vi "Launch Scoring Manager.vi"(8 "error in (no error)":errorcluster, 11 "SOL-Server in":refnum<class "SOL-Server.lvclass">) -> (0 "error out":errorcluster, 3 "SOL-Server out":refnum<class "SOL-Server.lvclass">)   [LabVIEW 2020, in "Summer of LabVIEW.lvlib" / "SOL-Server.lvclass"]
uses:
  SOL-Server.lvclass
  Scoring Manager Async.vi
  SOL-Server.lvclass/SOL-Server.ctl
  SOL-Config/SOL-Config.lvclass
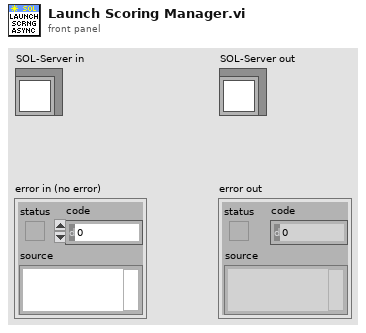
[diagram p1: front panel]
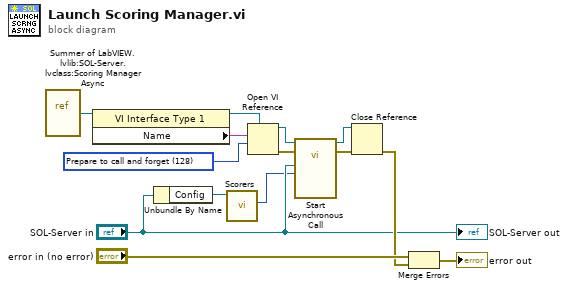
[diagram p0: block diagram]
diagram:
  w8 = 128 items=["Record modifications"=1, "Open templates for editing"=2, "Prompt user to save"=4, "Prepare for reentrant run"=8, "Prompt to find missing subVIs"=16, "Hide loading dialog box"=32, "Enable simultaneous calls"=64, "Prepare to call and forget"=128, "Simultaneous call and forget"=192, "Prepare to call and collect"=256, "Simultaneous call and collect"=320]
  n1 = vi-ref "Summer of LabVIEW.lvlib:SOL-Server.lvclass:Scoring Manager Async.vi"() -> (w6:refnum<vi>)
  n2 = property class="VI Interface Type 1"(reference=w6) -> (reference out=w9:refnum<vi>, "Name"=w7:string)  [unwired: 1 in, 1 out]
  n3 = Unbundle By Name("SOL-Server in") -> ("Config"=w2:refnum<class "SOL-Config.lvclass">)
  n4 = call "Scorers.vi"("SOL-Config in"=w2) -> ("Scorers"=w1:i32)  [unwired: 8 in, 2 out]
  n5 = Open VI Reference(type specifier VI Refnum (for type only)=w9, vi path=w7, options=w8) -> (vi reference=w11:refnum<vi>, error out=w10:errorcluster)  [unwired: 3 in]
  n6 = call-by-ref "Start Asynchronous Call"(reference=w11, error in=w10, "Pool Size (2)"=w1, "SOL-Server in"="SOL-Server in") -> (reference out=w13:refnum<vi>, error out=w12:errorcluster)  [unwired: 10 in]
  n7 = Close Reference(reference=w13, error in (no error)=w12) -> (error out=w4:errorcluster)
  n8 = Merge Errors("error in (no error)", w4) -> (→"error out":errorcluster)
  "SOL-Server out" <- "SOL-Server in"
